vi "Get Object (RAW data).vi"(6 "Version ID":string, 7 "Request Parameters":T1, 8 "error in (no error)":errorcluster, 9 "Bucket":string, 10 "Path":string) -> (0 "error out":errorcluster, 2 "GetObjectResult":T3, 3 "Data":string)   [LabVIEW 2011, in "LV Interface for Amazon S3.lvlib"]
doc: "This operation <B>retrieves an object</B> from Amazon S3 <B> and returns RAW data. You must have READ access</B> to the object. If you grant READ access to the anonymous user, you can return the object without using an authorization header. To distribute large files to many people, you can <B>save bandwidth costs using BitTorrent</B>. You can <B>limit returned data using Request parameters</B>."
uses:
  LV Interface for Amazon S3.lvlib
  Typedefs/AMZ_S3_API_GETObjectResult.ctl
  Typedefs/AMZ_S3_API_GET Object Request Parameters.ctl
  Typedefs/AMZ_S3_API_GET Request Range.ctl
  Typedefs/AMZ_S3_Call Results.ctl
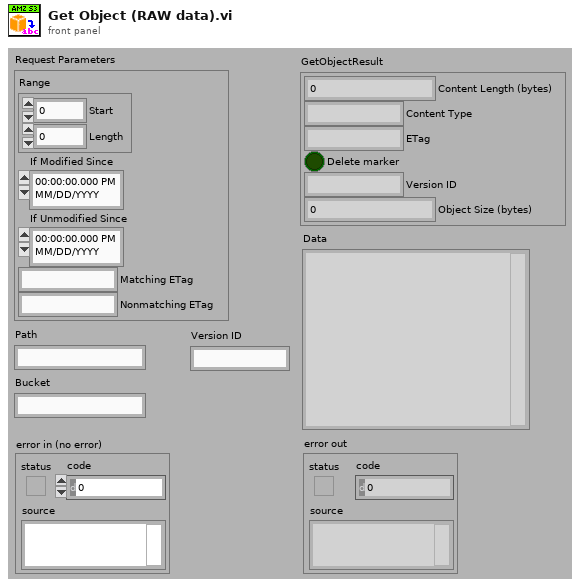
[diagram p1: front panel]
types:
  T1 = typedef "LV Interface for Amazon S3.lvlib/AMZ_S3_API_GET Object Request Parameters.ctl" = cluster{"Range":T2, "If Modified Since":timestamp, "If Unmodified Since":timestamp, "Matching ETag":string, "Nonmatching ETag":string}
  T2 = typedef "LV Interface for Amazon S3.lvlib/AMZ_S3_API_GET Request Range.ctl" = cluster{"Start":i64, "Length":i64}
  T3 = typedef "LV Interface for Amazon S3.lvlib/AMZ_S3_API_GETObjectResult.ctl" = cluster{"Content Length (bytes)":u64, "Content Type":string, "ETag":string, "Delete marker":bool, "Version ID":string, "Object Size (bytes)":u64}
  T4 = typedef "LV Interface for Amazon S3.lvlib/AMZ_S3_Call Results.ctl" = enum16{"Success", "UndefinedError", "AccessDenied", "AccountProblem", "AmbiguousGrantByEmailAddress", "BadDigest", "BucketAlreadyExists", "BucketAlreadyOwnedByYou", "BucketNotEmpty", "CredentialsNotSupported", "CrossLocationLoggingProhibited", "EntityTooSmall", "EntityTooLarge", "ExpiredToken", "IllegalVersioningConfigurationException", "IncompleteBody", "IncorrectNumberOfFilesInPostRequest", "InlineDataTooLarge", "InternalError", "InvalidAccessKeyId", "InvalidAddressingHeader", "InvalidArgument", "InvalidBucketName", "InvalidDigest", "InvalidLocationConstraint", "InvalidPart", "InvalidPartOrder", "InvalidPayer", "InvalidPolicyDocument", "InvalidRange", "InvalidSecurity", "InvalidSOAPRequest", "InvalidStorageClass", "InvalidTargetBucketForLogging", "InvalidToken", "InvalidURI", "KeyTooLong", "MalformedACLError", "MalformedPOSTRequest", "MalformedXML", "MaxMessageLengthExceeded", "MaxPostPreDataLengthExceededError", "MetadataTooLarge", "MethodNotAllowed", "MissingAttachment", "MissingContentLength", "MissingRequestBodyError", "MissingSecurityElement", "MissingSecurityHeader", "NoLoggingStatusForKey", "NoSuchBucket", "NoSuchKey", "NoSuchUpload", "NoSuchVersion", "NotImplemented", "NotSignedUp", "OperationAborted", "PermanentRedirect", "PreconditionFailed", "Redirect", "RequestIsNotMultiPartContent", "RequestTimeout", "RequestTimeTooSkewed", "RequestTorrentOfBucketError", "SignatureDoesNotMatch", "SlowDown", "TemporaryRedirect", "TokenRefreshRequired", "TooManyBuckets", "UnexpectedContent", "UnresolvableGrantByEmailAddress", "UserKeyMustBeSpecified", "LabVIEWError"}
  T5 = typedef "LV Interface for Amazon S3.lvlib/AMZ_S3_HTTP Header-Value pair.ctl" = cluster{"Header":string, "Value":string}
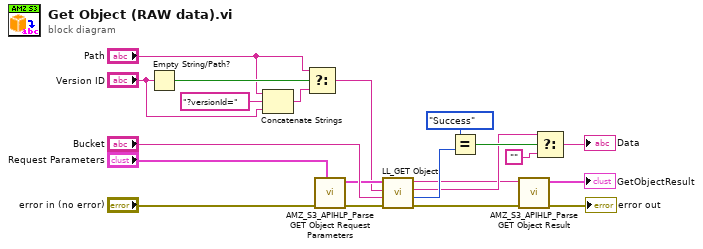
[diagram p0: block diagram]
diagram:
  n1 = Empty String/Path?(string/path="Version ID") -> (empty?=w10:bool)
  n2 = Concatenate Strings("Path", "?versionId=" ("string"), "Version ID") -> (w6:string)
  n3 = Select(t="Path", s=w10, f=w6) -> (s? t:f=w5:string)
  n4 = call "AMZ_S3_APIHLP_Parse GET Object Request Parameters.vi"("GET Object Request Parameters"="Request Parameters", "error in (no error)"="error in (no error)") -> ("error out"=w20:errorcluster, "HTTP Headers"=w19:T5[])  [unwired: 8 in]
  n5 = call "LL_GET Object.vi"("error in (no error)"=w20, "Bucket"="Bucket", "Path and query string"=w5, "Headers"=w19) -> ("error out"=w4:errorcluster, "Call Result"=w16:T4, "Response body"=w13:string, "Response header"=w3:string)  [unwired: 4 in]
  n6 = Equal?(x=AMZ_S3_Call_Results."Success" ("y"), y=w16) -> (x = y?=w14:bool)
  n7 = call "AMZ_S3_APIHLP_Parse GET Object Result.vi"("error in (no error)"=w4, "Response header"=w3) -> ("error out"=→"error out":errorcluster, "GetObjectResult"=→"GetObjectResult":T3)  [unwired: 8 in]
  n8 = Select(t=w13, s=w14, f="") -> (s? t:f=→"Data":string)
